vi "Create - Random Signal.vi"(0 "reference in":refnum<class "GSwFormDSP.lvclass">, 5 "error in (no error)":errorcluster) -> (14 "reference in":refnum<class "GSwFormDSP.lvclass">, 19 "error out":errorcluster)   [LabVIEW 2020, in "GSwFormDSP.lvclass"]
uses:
  GSwFormDSP.lvclass
  <vilib>/Analysis/NI_AALBase.lvlib
panel:
  in  "Done":bool
  in  "Duration (s)":dbl=10.0 min=1.0 max=3600.0 step=0.1 format="%.1f"
  in  "User Input Fs":T1(ring)=enum."44100 Hz" caption="Sampling Rate"
  in  "Amplitude":dbl=1.0 format="%.2f"
  in  "Signal Name":string="unknown"
  in  "Signal Unit":string="unknown"
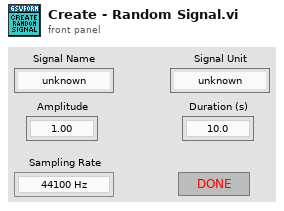
[diagram p1: front panel]
types:
  T1 = enum16{"256 Hz", "512 Hz", "1024 Hz", "2048 Hz", "4096 Hz", "8192 Hz", "11025 Hz", "16384 Hz", "22050 Hz", "32768 Hz", "44100 Hz"}
  T2 = enum16{"Replace Current Signals", "Append to Current Signals"}
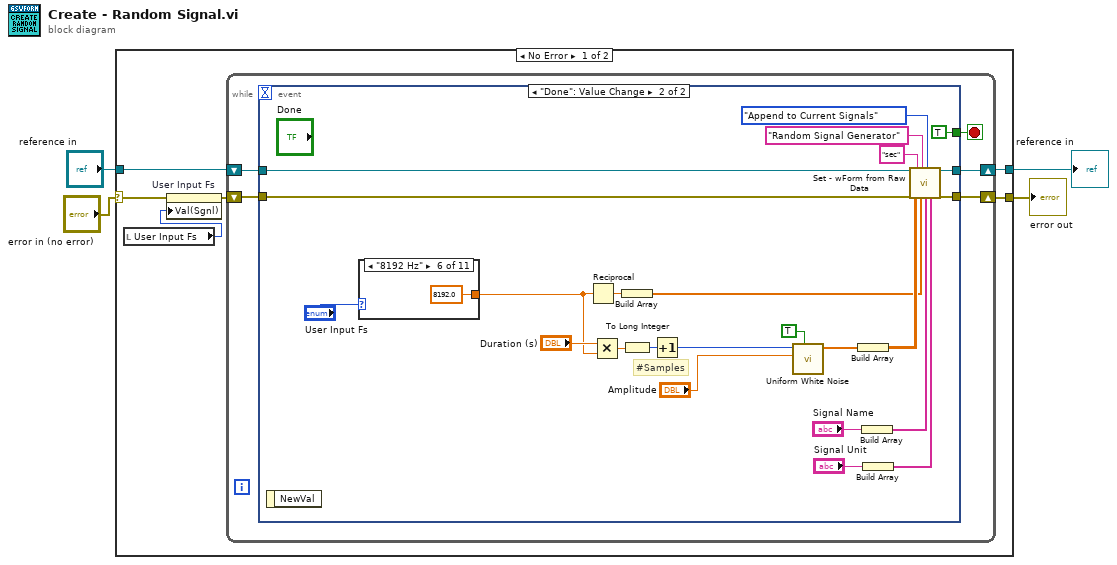
[diagram p0: block diagram]
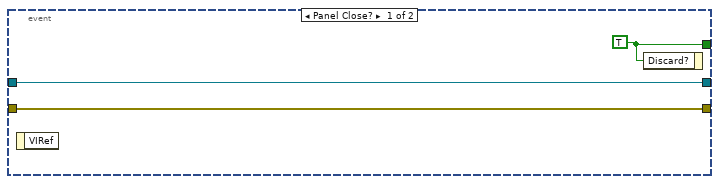
[diagram p2: hidden frame]
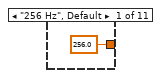
[diagram p3: hidden frame]
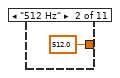
[diagram p4: hidden frame]
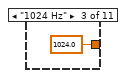
[diagram p5: hidden frame]
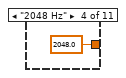
[diagram p6: hidden frame]
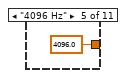
[diagram p7: hidden frame]
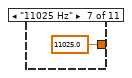
[diagram p8: hidden frame]
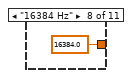
[diagram p9: hidden frame]
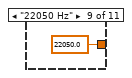
[diagram p10: hidden frame]
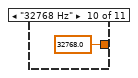
[diagram p11: hidden frame]
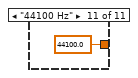
[diagram p12: hidden frame]
diagram:
  n1 = case shown="No Error" "error in (no error)" {
    selector: "error in (no error)" -> [w5 w55]
    tunnel: [w8 w55] -> w3
    tunnel: [w9 w54] -> w1
    tunnel: "reference in" -> [w10 w54]
    frame No Error {
      n2 = local read "User Input Fs"() -> (w6:T1)
      n3 = property on="User Input Fs" class="Enum (strict)"(error in=w5, "Val(Sgnl)"=w6) -> (error out=w7:errorcluster)  [unwired: 1 in, 1 out]
      n4 = while {
        shift-right: [w13] -> w9
        shift-left: w10 -> [w14]
        shift-right: [w12] -> w8
        shift-left: w7 -> [w11]
        stop <- w15 stop-if-true
        n5 = event shown="[1] \"Done\": Value Change" {
          selector: _ -> [_ _]
          dyn-events: _ -> [_ _]
          timeout: _ -> [_ _]
          tunnel: [w18 TRUE ("Discard?")] -> w15
          tunnel: w14 -> [w17 w29]
          tunnel: [w17 w28] -> w13
          tunnel: [w16 w27] -> w12
          tunnel: w11 -> [w16 w26]
          event Panel Close? {
            w18 = TRUE ("Discard?")
            n6 = event-data() -> ()  [unwired: 1 in, 1 out]
            n7 = event-data("Discard?"=w18) -> ()  [unwired: 1 in, 1 out]
          }
          event "Done": Value Change {
            # "#Samples"
            n8 = event-data() -> ()  [unwired: 1 in, 1 out]
            n9 = case shown="\"8192 Hz\"" "User Input Fs" {
              tunnel: [256.0 512.0 1024.0 2048.0 4096.0 8192.0 11025.0 16384.0 22050.0 32768.0 44100.0] -> w23
              frame "256 Hz", Default {
              }
              frame "512 Hz" {
              }
              frame "1024 Hz" {
              }
              frame "2048 Hz" {
              }
              frame "4096 Hz" {
              }
              frame "8192 Hz" {
              }
              frame "11025 Hz" {
              }
              frame "16384 Hz" {
              }
              frame "22050 Hz" {
              }
              frame "32768 Hz" {
              }
              frame "44100 Hz" {
              }
            }
            n10 = Reciprocal(x=w23) -> (1/x=w39:dbl)
            n11 = Multiply(x="Duration (s)", y=w23) -> (x*y=w41:dbl)
            n12 = Build Array(w39) -> (w35:dbl[])
            n13 = To Long Integer(number=w41) -> (32bit integer=w40:i32)
            n14 = Increment(x=w40) -> (x+1=w22:i32)
            n15 = call <vilib>:"Uniform White Noise.vi"("initialize?"=TRUE, "amplitude"="Amplitude", "samples"=w22) -> ("uniform white noise"=w19:dbl[])  [unwired: 7 in, 1 out]
            n16 = Build Array(w19) -> (w36:dbl[][])
            n17 = Build Array("Signal Name") -> (w34:string[])
            n18 = Build Array("Signal Unit") -> (w33:string[])
            n19 = call "Set - wForm from Raw Data.vi"("reference in"=w29, "error in (no error)"=w26, "X Unit"="sec", "Y Data (Row matrix)"=w36, "Data Origin"="Random Signal Generator", "dTs"=w35, "Signal Set"=T2."Append to Current Signals", "Signals Name"=w34, "Signals Unit"=w33) -> ("reference in"=w28:refnum<class "GSwFormDSP.lvclass">, "error out"=w27:errorcluster)  [unwired: 9 in]
          }
        }
      }
    }
    frame Error {
    }
  }
  "error out" <- w3
  "reference in" <- w1
